vi "Write Test Report.vi"(10 "Test Report":refnum<class "Test Report.lvclass">, 11 "Test Manager in":refnum<class "Test Manager.lvclass">) -> (3 "Test Manager out":refnum<class "Test Manager.lvclass">)   [LabVIEW 2013, in "Caraya.lvlib" / "Test Manager.lvclass"]
uses:
  Test Manager.lvclass
  Test Report/Test Report.lvclass
  Test Manager.lvclass/Test Manager.ctl
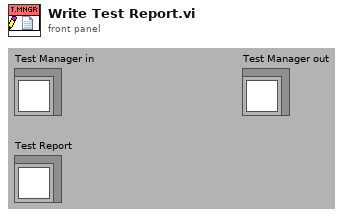
[diagram p1: front panel]
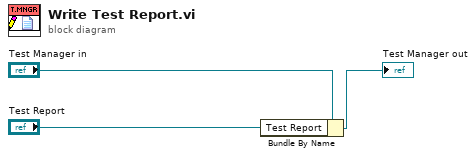
[diagram p0: block diagram]
diagram:
  n1 = Bundle By Name(cluster="Test Manager in", "Test Report"="Test Report") -> (→"Test Manager out":refnum<class "Test Manager.lvclass">)
